vi "CODCr电源命令.vi"(10 "通电/断电":bool, 11 "队列":refnum<queue>) -> (3 "队列输出":refnum<queue>)   [LabVIEW 2016, in "PLC.lvlib"]
uses:
  PLC.lvlib
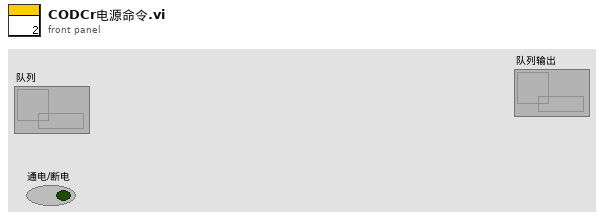
[diagram p1: front panel]
types:
  T1 = cluster{"命令":string, "data":cluster{"starting address":u16, "coil values":bool[]}}
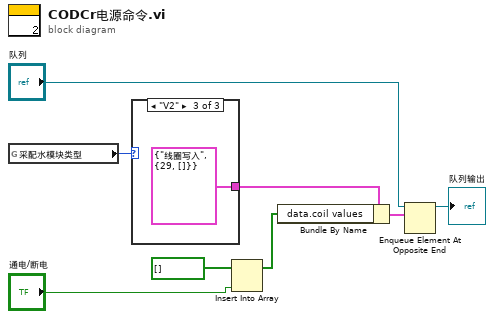
[diagram p0: block diagram]
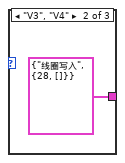
[diagram p3: hidden frame]
diagram:
  n1 = global read "系统设置全局变量.vi" "采配水模块类型"() -> (w2:enum16{"V1", "V2", "V3", "V4", "室内V1", "室内V2"})
  n2 = case shown="\"V2\"" w2 {
    tunnel: [_ T1 {"命令"="线圈写入", "data"={"starting address"=28, "coil values"=[]}} ("元素") T1 {"命令"="线圈写入", "data"={"starting address"=29, "coil values"=[]}} ("元素")] -> w1
    frame "V1", Default {
    }
    frame "V3", "V4" {
    }
    frame "V2" {
    }
  }
  n3 = Insert Into Array(array=bool[] [] ("data.coil values"), new element="通电/断电") -> (w4:bool[])  [unwired: 1 in]
  n4 = Bundle By Name(cluster=w1, "data.coil values"=w4) -> (w8:T1)
  n5 = Enqueue Element At Opposite End(queue="队列", element=w8) -> (queue out=→"队列输出":refnum<queue>)  [unwired: 2 in, 2 out]
